vi "AVS_GetSaturatedPixels.vi"(0 "a_hDevice":i32, 7 "a_pSaturated":u8[](array[numeric])) -> (4 "Output Value":i32, 8 "a_pSaturated":u8[](array[numeric]))   [LabVIEW 2013, in "AvaSpec.lvlib" / "Avantes Spectrometer Functions.lvlib"]
uses:
  Avantes Spectrometer Functions.lvlib
  polling_mc/AS5216.dll
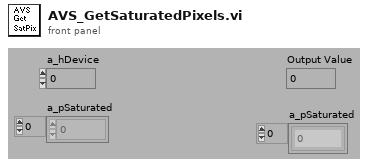
[diagram p1: front panel]
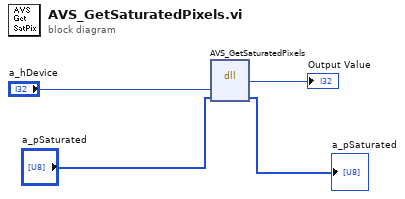
[diagram p0: block diagram]
diagram:
  n1 = dll-call lib="C:/Users/dhstuart/Dropbox/CLTC/avantesSpectrometer/Libraries/AS-5216-DLL/polling_mc/AS5216.dll" fn="AVS_GetSaturatedPixels"("a_hDevice"="a_hDevice", "a_pSaturated"="a_pSaturated") -> ("return type"=→"Output Value":i32, "a_pSaturated"=→"a_pSaturated":u8[])  [unwired: 4 in, 2 out]
